vi "[GV]_GPS Stop.vi"() -> ()   [LabVIEW 2016]
panel:
  in  "GPS Stop":bool
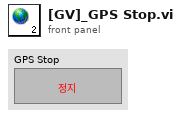
[diagram p1: front panel]
diagram:
